vi "PROXY_hex_whitespace_in_diagnostic_messages.vi"(11 "message_history":T1[](array[typedef])) -> (3 "hexed_records":string[][](array[string]))   [LabVIEW 2020]
uses:
  FGV/DIAGNOSTICS_message_history_buffer/PROXY_DIAGNOSTICS_message_history_buffer_all_info.ctl
  STATION/station.ctl
  _misc/DIAGNOSTICS_message_type.ctl
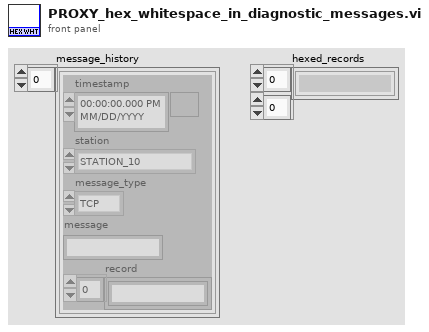
[diagram p1: front panel]
types:
  T1 = typedef "PROXY_DIAGNOSTICS_message_history_buffer_all_info.ctl" = cluster{"timestamp":timestamp, "station":T2, "message_type":T3, "message":string, "record":string[]}
  T2 = typedef "station.ctl" = enum16{"STATION_10", "STATION_20", "STATION_30", "STATION_40", "STATION_50", "STATION_60", "STATION_70", "STATION_80", "STATION_90", "STATION_100", "STATION_110", "STATION_120", "STATION_165", "MAIN"}
  T3 = typedef "DIAGNOSTICS_message_type.ctl" = enum16{"TCP", "SQL"}
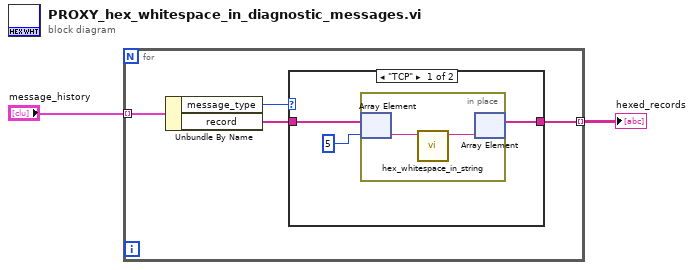
[diagram p0: block diagram]
diagram:
  n1 = for {
    tunnel: "message_history" -> [w6] mode=indexing
    tunnel: [w3] -> w2 mode=indexing
    n2 = Unbundle By Name(w6) -> ("message_type"=w5:T3, "record"=w4:string[])
    n3 = case shown="\"TCP\"" w5 {
      tunnel: w4 -> [w9 w12]
      tunnel: [w8 w12] -> w3
      frame "TCP" {
        n4 = in-place {
          n5 = in-place-array #1(w9, 5) -> (w11:string)
          n6 = call "hex_whitespace_in_string.vi"("string"=w11) -> ("hexed_string"=w10:string)  [unwired: 10 in]
          n7 = in-place-array #1(w10) -> (w8:string[])  [unwired: 1 out]
        }
      }
      frame "SQL" {
      }
    }
  }
  "hexed_records" <- w2
